vi "area_triangulo.vi"() -> ()   [LabVIEW 2013]
panel:
  in  "stop":bool
  out "Área (cm²)":dbl
  in  "Base (cm)":dbl
  in  "Altura (cm)":dbl
  # "Área do Triangulo"
  # "<------  Altura ----->"
  # "<--------  Base ------->"
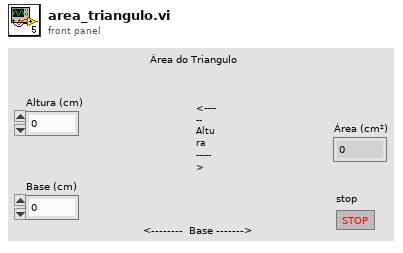
[diagram p1: front panel]
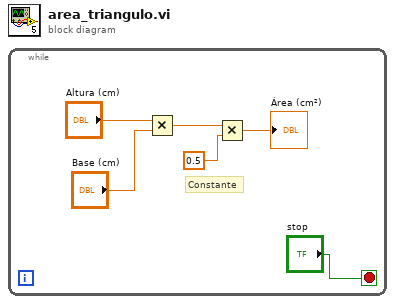
[diagram p0: block diagram]
diagram:
  n1 = while {
    stop <- "stop" stop-if-true
    # "Constante"
    n2 = Multiply(x="Altura (cm)", y="Base (cm)") -> (x*y=w5:dbl)
    n3 = Multiply(x=w5, y=0.5) -> (x*y=→"Área (cm²)":dbl)
  }
